vi "counter_event_v3.vi"() -> ()   [LabVIEW 2019]
panel:
  in  "Reset":bool
  in  "stop":bool
  out "Count":u32
  in  "Button":bool
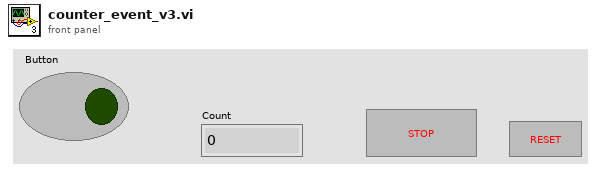
[diagram p1: front panel]
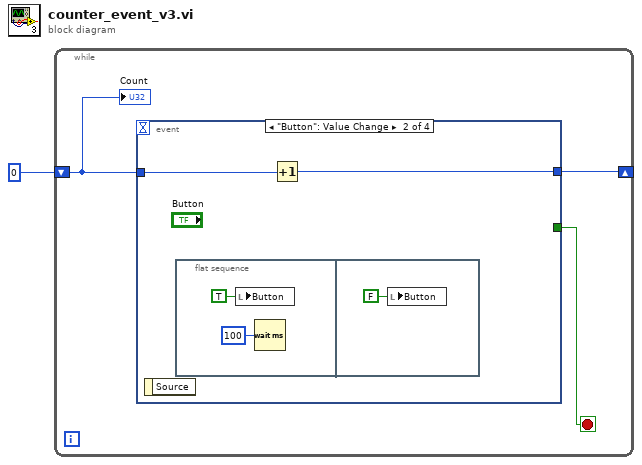
[diagram p0: block diagram]
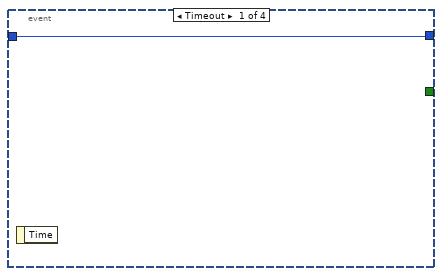
[diagram p2: hidden frame]
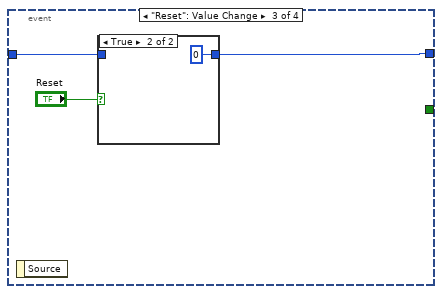
[diagram p3: hidden frame]
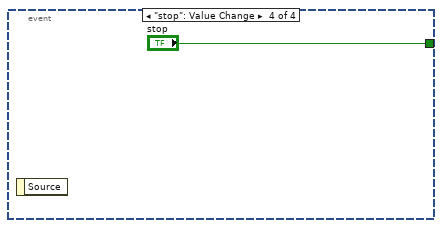
[diagram p5: hidden frame]
diagram:
  n1 = while {
    shift-right: [w3] -> _
    shift-left: u32 0 ("milliseconds to wait") -> [w4]
    stop <- w2 stop-if-true
    n2 = event shown="[1] \"Button\": Value Change" {
      selector: _ -> [_ _ _ _]
      dyn-events: _ -> [_ _ _ _]
      timeout: _ -> [_ _ _ _]
      tunnel: w4 -> [w5 w7 w12 _]
      tunnel: [w5 w6 w11 _] -> w3
      tunnel: [_ _ _ "stop"] -> w2
      event Timeout {
        n3 = event-data() -> ()  [unwired: 1 in, 1 out]
      }
      event "Button": Value Change {
        n4 = event-data() -> ()  [unwired: 1 in, 1 out]
        n5 = flat-sequence {
          frame #0 {
            n6 = local write "Button"(TRUE ("Button")) -> ()
            n7 = Wait (ms)(milliseconds to wait=u32 100) -> ()  [unwired: 1 out]
          }
          frame #1 {
            n8 = local write "Button"(FALSE ("Button")) -> ()
          }
        }
        n9 = Increment(x=w7) -> (x+1=w6:u32)
      }
      event "Reset": Value Change {
        n10 = event-data() -> ()  [unwired: 1 in, 1 out]
        n11 = case shown="True" "Reset" {
          tunnel: w12 -> [w14 _]
          tunnel: [w14 u32 0 ("milliseconds to wait")] -> w11
          frame False {
          }
          frame True {
          }
        }
      }
      event "stop": Value Change {
        n12 = event-data() -> ()  [unwired: 1 in, 1 out]
      }
    }
    "Count" <- w4
  }
